vi "Render.vi"(10 "Destination":T1, 11 "Texture in":refnum<class "Texture.lvclass">) -> ()   [LabVIEW 2015, in "Texture.lvclass"]
uses:
  Texture.lvclass
  LabSDL2/Source/Libraries/SDL2 Utility/Point (I32).ctl
  Texture.lvclass/Texture.ctl
  LabSDL2/Source/Libraries/LibSDL2 Wrapper/Controls/NULL.ctl
  LabSDL2/Source/Libraries/LibSDL2 Wrapper/Controls/Rectangle.ctl
  Globals.vi
  LabSDL2/Source/Libraries/LibSDL2 Wrapper/LibSDL2.lvlib
  LabSDL2/Source/Libraries/SDL2 Utility/SDL2 Utility.lvlib
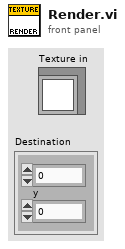
[diagram p1: front panel]
types:
  T1 = typedef "SDL2 Utility.lvlib/Point (I32).ctl" = cluster{"x":i32, "y":i32}
  T2 = typedef "LibSDL2.lvlib/Rectangle.ctl" = cluster{"x":i32, "y":i32, "Width":i32, "Height":i32}
  T3 = typedef "LibSDL2.lvlib/NULL.ctl" = enum32{"NULL"}
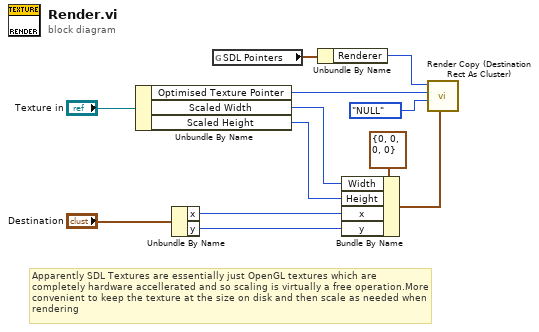
[diagram p0: block diagram]
diagram:
  # "Apparently SDL Textures are essentially just OpenGL textures which are completely hardware accellerated and so scaling is virtually a free operation.More convenient to keep the texture at the size on disk and then scale as needed when rendering"
  n1 = Unbundle By Name("Texture in") -> ("Optimised Texture Pointer"=w3:u32, "Scaled Width"=w2:i32, "Scaled Height"=w1:i32)
  n2 = Unbundle By Name("Destination") -> ("x"=w11:i32, "y"=w12:i32)
  n3 = global read "Globals.vi" "SDL Pointers"() -> (w5:cluster{"Renderer":u32, "Font":u32})
  n4 = Unbundle By Name(w5) -> ("Renderer"=w4:u32)
  n5 = Bundle By Name(cluster=T2 {"x"=0, "y"=0, "Width"=0, "Height"=0} ("Destination Rectangle"), "Width"=w2, "Height"=w1, "x"=w11, "y"=w12) -> (w10:T2)
  n6 = call "Render Copy (Destination Rect As Cluster).vi"("Destination Rectangle"=w10, "Source Rectangle Pointer"=NULL."NULL" ("Null"), "Texture Pointer"=w3, "Renderer Pointer"=w4) -> ()  [unwired: 7 in, 1 out]
